vi "BlockInfo.vi"() -> ()   [LabVIEW 2015]
uses:
  lib/Snap7.lvlib
panel:
  out "?":string
  in  "stop":bool
  out "Struct Info":T1 {"Chksum" format="%x"; "Version" format="%x"}
  in  "BlockNumber":i32
  in  "BlockType":i32(ring)=68 items=["OB"=56, "DB"=65, "SDB"=66, "FC"=67, "SFC"=68, "FB"=69, "SFB"=70]
  out "Status":string
  out "Header":string
  out "Family":string
  out "Author":string
  out "Interface Date":string
  out "Code Date":string
  in  "Slot":i32=2
  in  "Rack":i32
  in  "Address IP":string="192.168.1.12"
  # "Creation Info"
  # "For BlkType and BlkLang legenda see snap7.h"
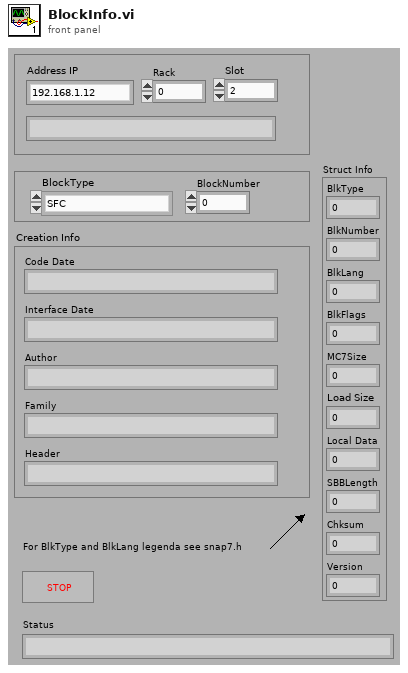
[diagram p1: front panel]
types:
  T1 = cluster{"BlkType":i32, "BlkNumber":i32, "BlkLang":i32, "BlkFlags":i32, "MC7Size":i32, "Load Size":i32, "Local Data":i32, "SBBLength":i32, "Chksum":i32, "Version":i32}
  T2 = cluster{"BlkType":i32, "BlkNumber":i32, "BlkLang":i32, "BlkFlags":i32, "MC7Size":i32, "Load Size":i32, "Local Data":i32, "SBB Length":i32, "Chksum":i32, "Version":i32}
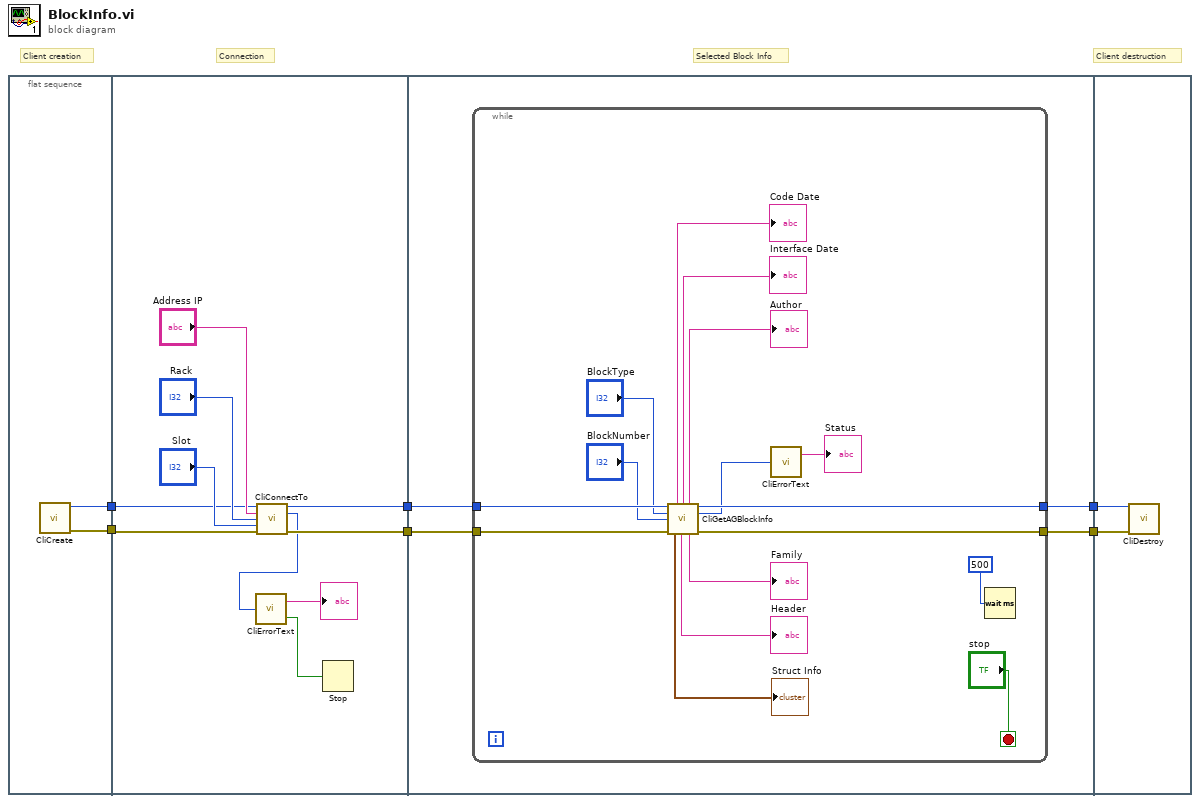
[diagram p0: block diagram]
diagram:
  # "Selected Block Info"
  # "Client destruction"
  # "Connection"
  # "Client creation"
  n1 = flat-sequence {
    tunnel: [w8] -> w4
    tunnel: [w7] -> w3
    tunnel: [w18] -> w6
    tunnel: [w12] -> w5
    tunnel: w4 -> [w14]
    tunnel: w3 -> [w13]
    tunnel: w6 -> [w22]
    tunnel: w5 -> [w21]
    tunnel: [w20] -> w2
    tunnel: [w19] -> w1
    tunnel: w2 -> [w40]
    tunnel: w1 -> [w39]
    frame #0 {
      n2 = call "CliCreate.vi"() -> ("ref out"=w8:u64, "error out"=w7:errorcluster)  [unwired: 14 in]
    }
    frame #1 {
      n3 = call "CliConnectTo.vi"("ref in"=w14, "Address"="Address IP", "Rack"="Rack", "Slot"="Slot", "error in (no error)"=w13) -> ("ref out"=w12:u64, "Result"=w9:i32, "error out"=w18:errorcluster)  [unwired: 8 in]
      n4 = call "CliErrorText.vi"("ErrNo"=w9) -> ("Error"=w11:bool, "ErrMessage"=→"?":string)
      n5 = Stop(stop? (T)=w11) -> ()
    }
    frame #2 {
      n6 = while {
        tunnel: w22 -> [w38]
        tunnel: w21 -> [w37]
        tunnel: [w36] -> w20
        tunnel: [w35] -> w19
        stop <- "stop" stop-if-true
        n7 = call "CliGetAGBlockInfo.vi"("ref in"=w37, "BlockType"="BlockType", "BlockNumber"="BlockNumber", "error in (no error)"=w38) -> ("Code Date"=→"Code Date":string, "Interface Date"=→"Interface Date":string, "Author"=→"Author":string, "ref out"=w36:u64, "Result"=w24:i32, "IntInfo"=→"Struct Info":T2, "Header"=→"Header":string, "Family"=→"Family":string, "error out"=w35:errorcluster)  [unwired: 3 in]
        n8 = call "CliErrorText.vi"("ErrNo"=w24) -> ("ErrMessage"=→"Status":string)  [unwired: 1 out]
        n9 = Wait (ms)(milliseconds to wait=u32 500 ("Loop Delay (ms)")) -> ()  [unwired: 1 out]
      }
    }
    frame #3 {
      n10 = call "CliDestroy.vi"("ref in"=w40, "error in (no error)"=w39) -> ()  [unwired: 13 in, 1 out]
    }
  }
